vi "Tree.vi"   [LabVIEW 2016, in "Instrument.VNA.lvclass"]
uses:
  Instrument.VNA.lvclass
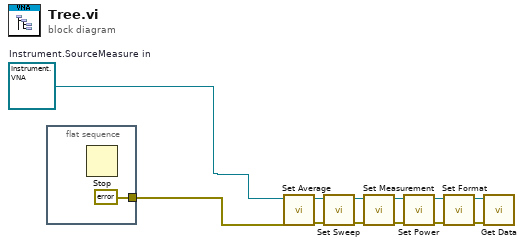
[diagram p0: block diagram]
diagram:
  w11 = refnum<class "Instrument.VNA.lvclass"> refnum  # Instrument.SourceMeasure in
  n1 = flat-sequence {
    tunnel: [errorcluster {"status"=FALSE, "code"=0, "source"=""} ("error in (no error)")] -> w12
    frame #0 {
      n2 = Stop() -> ()  [unwired: 1 in]
    }
  }
  n3 = call-dynamic "Set Average.vi"("error in (no error)"=w12, "Instrument.VSource in"=w11) -> ("error out"=w9:errorcluster, "Instrument.VSource out"=w10:refnum<class "Instrument.VNA.lvclass">)  [unwired: 8 in]
  n4 = call-dynamic "Set Sweep.vi"("error in (no error)"=w9, "Instrument.VSource in"=w10) -> ("error out"=w7:errorcluster, "Instrument.VSource out"=w8:refnum<class "Instrument.VNA.lvclass">)  [unwired: 8 in]
  n5 = call-dynamic "Set Measurement.vi"("error in (no error)"=w7, "Instrument.VSource in"=w8) -> ("error out"=w5:errorcluster, "Instrument.VSource out"=w6:refnum<class "Instrument.VNA.lvclass">)  [unwired: 8 in]
  n6 = call-dynamic "Set Power.vi"("error in (no error)"=w5, "Instrument.VSource in"=w6) -> ("error out"=w3:errorcluster, "Instrument.VSource out"=w4:refnum<class "Instrument.VNA.lvclass">)  [unwired: 8 in]
  n7 = call-dynamic "Set Format.vi"("error in (no error)"=w3, "Instrument.VSource in"=w4) -> ("error out"=w1:errorcluster, "Instrument.VSource out"=w2:refnum<class "Instrument.VNA.lvclass">)  [unwired: 8 in]
  n8 = call-dynamic "Get Data.vi"("error in (no error)"=w1, "Instrument.VSource in"=w2) -> ()  [unwired: 7 in, 3 out]
